vi "grabSetup_action.vi"(0 "HGF_ImaqUsb":refnum<class "HGF_ImaqUsb.lvclass">, 5 "error in (no error)":errorcluster, 6 "Region of Interest":i32[](array[numeric]), 7 "Step x":i32=-1, 8 "Channel":i32=-1, 9 "Step y":i32=-1) -> (14 "dup HGF_ImaqUsb":refnum<class "HGF_ImaqUsb.lvclass">, 19 "error out":errorcluster)   [LabVIEW 2009, in "HGF_ImaqUsb.lvclass"]
doc: "Starts a grab acquisition. This VI performs a continuous acquisition that provides access to the most recently acquired image.\n\nParameter are used for framegrabber, only, and can be ignored for IMAQdx and IMAQ for USB."
uses:
  HGF_ImaqUsb.lvclass
  HGF_ImaqUsb.lvclass/HGF_ImaqUsb.ctl
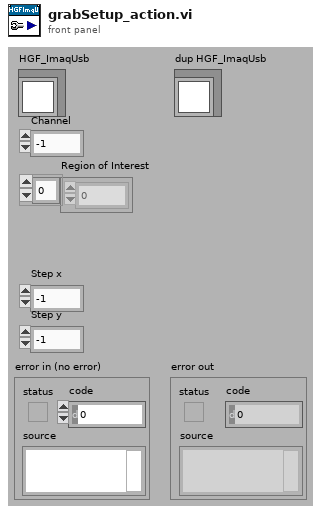
[diagram p1: front panel]
types:
  T1 = typedef "IMAQ USB.ctl" = refnum<k1>
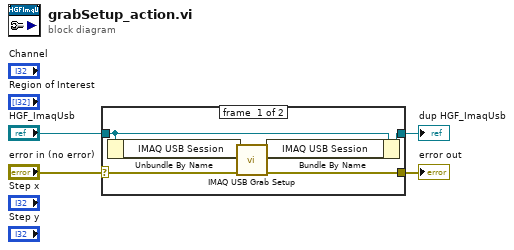
[diagram p0: block diagram]
diagram:
  n1 = case shown="No Error" "error in (no error)" {
    selector: "error in (no error)" -> [w5 w11]
    tunnel: "HGF_ImaqUsb" -> [w9 w12]
    tunnel: [w7 w12] -> w3
    tunnel: [w6 w11] -> w2
    frame #0 {
      n2 = Unbundle By Name(w9) -> ("IMAQ USB Session"=w10:T1)
      n3 = call <vilib>:"IMAQ USB Grab Setup.vi"("error in (no error)"=w5, "IMAQ USB Session In"=w10) -> ("error out"=w6:errorcluster, "IMAQ USB Session Out"=w8:T1)  [unwired: 8 out]
      n4 = Bundle By Name(cluster=w9, "IMAQ USB Session"=w8) -> (w7:refnum<class "HGF_ImaqUsb.lvclass">)
    }
    frame #1 {
    }
  }
  "error out" <- w2
  "dup HGF_ImaqUsb" <- w3
